vi "Distance from Acceleration, Time and Initial Velocity.vi"(0 "Initial Velocity (in/s)":dbl, 5 "Acceleration (in/s2)":dbl, 7 "Time (s)":dbl) -> (4 "Distance (in)":dbl, 6 "Final Velocity (in/s)":dbl)   [LabVIEW 2019, in "Motion Profile Generator.lvclass"]
uses:
  Motion Profile Generator.lvclass
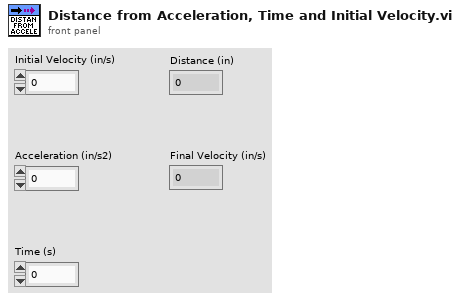
[diagram p1: front panel]
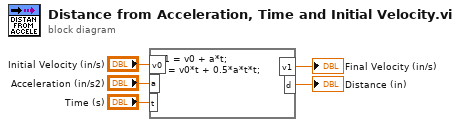
[diagram p0: block diagram]
diagram:
  n1 = formula code="v1 = v0 + a*t;\nd = v0*t + 0.5*a*t*t;"("v0"="Initial Velocity (in/s)", "a"="Acceleration (in/s2)", "t"="Time (s)") -> ("d"=→"Distance (in)":dbl, "v1"=→"Final Velocity (in/s)":dbl)
